vi "Main.vi"(11 "Module Admin":refnum<class "Delacor_lib_QMH_Module Admin.lvclass">) -> ()   [LabVIEW 2022 SP3, in "DBModule.lvlib"]
doc: "This template is based off of the Queued Message Handler design pattern and the Queued Message Handler project template that ships with LabVIEW.\n\nThe main difference is that the queue is private to this module and communication between modules is performed via Broadcast and Request events.\n\nRequest events are wrapped in public API methods and are handled in the Event Handling Loop (EHL) of this VI. Any module can register for Broadcast events sent by this module. The EHL generates messages based on user interface actions.\n\nThe Message Handling Loop (MHL) processes messages generated by the EHL, or by other messages. The messages are string values, so new messages can be added easily to the Message Cases case structure in the MHL. Each message cluster can also provide an optional value for Message Data, which is a variant that can be converted to whatever message-specific data is required.\n____\nHAMPEL SOFTWARE ENGINEERING v2.6.0 (2023-12-19 10:54)"
uses:
  DBModule.lvlib
  <vilib>/Delacor/Delacor QMH/Libraries/Module Admin_class/Delacor_lib_QMH_Module Admin.lvclass
  Module Data--cluster.ctl
  Libraries/hse-libraries/Source/hse-dqmh/Controls/Module Display Scenarios.ctl
  Stop Argument--cluster.ctl
  <vilib>/Delacor/Delacor QMH/Libraries/Message Queue_class/Delacor_lib_QMH_Message Queue.lvclass/Delacor_lib_QMH_Message Queue.ctl
  <vilib>/Delacor/Delacor QMH/Libraries/Module Admin_class/Delacor_lib_QMH_Module Admin.lvclass/Delacor_lib_QMH_Module Admin.ctl
  Configure Argument--cluster.ctl
  Prepare Argument--cluster.ctl
  Request UI Display Argument--cluster.ctl
  Request UI Display (Reply Payload)--cluster.ctl
  Libraries/hse-db/Source/DB-Engines/DB-SQLite/DB-SQLite.lvclass
  C:/Projects/579-Intelligent-Systems-Term-Project/06_Source/UI/FReVSys_Source/Libraries/hse-db/Source/DB-Interface/DB-Interface.lvclass
  <vilib>/Utility/miscctls.llb/LVPointTypeDef.ctl
  <vilib>/Delacor/Delacor QMH/Libraries/Message Queue_class/Delacor_lib_QMH_Enqueue Message (Single).vi
  <vilib>/Delacor/Delacor QMH/Libraries/Module Admin_class/Delacor_lib_QMH_Get External Launch.vi
  <vilib>/Utility/error.llb/Error Cluster From Error Code.vi
  <vilib>/ErrorRing/Error Ring.xnode
  <vilib>/Delacor/Delacor QMH/Libraries/Message Queue_class/Delacor_lib_QMH_Message Queue.lvclass
  Libraries/hse-libraries/Source/hse-configuration/config-ini/config-ini.lvclass
  <vilib>/Hampel Software Engineering/HSE Logger/hse-logger.lvlib
  Libraries/hse-libraries/Source/hse-dqmh/hse-dqmh.lvlib
  Libraries/hse-db/Source/DB_CONNECTOR/DB_CONNECTOR.lvlib
panel:
  in  "Names in DB":string[](array[string])
  in  "Write Names to DB":bool
  in  "Read Names from DB":bool
  out "DB-Engine":string
  out "Status DBC.":string caption="Status of DB_CONNECTOR"
  out "error out":errorcluster
  # "The \"DB Module\" serves as an example of how to use our HSE DB libraries.\n\nThe configuration file of this module (DBModule.ini) points towards the config section to be used in the \nDB_CONNECTOR module's config file (DB_CONNECTOR.ini).\n\nThe module then starts a clone of the DB_CONNECTOR module which it uses to access the SQLite db file.\n\nYou can use the buttons below to read from or write to a `test` table, and the status indicator below re-\ncreates the status display of the DB_CONNECTOR's API tester."
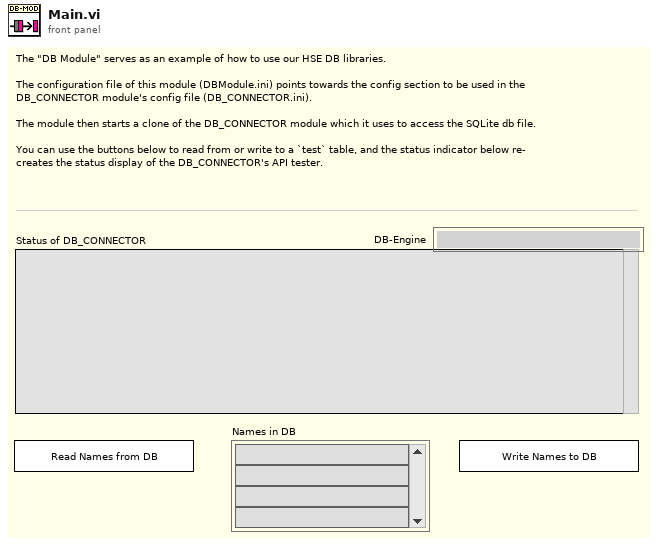
[diagram p1: front panel]
types:
  T1 = typedef "hse-db.lvlib/DB_CONNECTOR.lvlib/Broadcast Events--cluster.ctl" = cluster{"Module Did Init":refnum<user-event>, "Status Updated":refnum<user-event>, "Error Reported":refnum<user-event>, "Module Did Stop":refnum<user-event>, "Update Module Execution Status":refnum<user-event>, "Fast Query Reply":refnum<user-event>, "Configured and Connected":refnum<user-event>}
  T2 = typedef "DBModule.lvlib/Request Events--cluster.ctl" = cluster{"Stop Module":refnum<user-event>, "Show Panel":refnum<user-event>, "Hide Panel":refnum<user-event>, "Get Module Execution Status":refnum<user-event>, "Show Diagram":refnum<user-event>, "Configure":refnum<user-event>, "Prepare":refnum<user-event>, "Request UI Display":refnum<user-event>, "Start and Configure DB_Connector":refnum<user-event>}
  T3 = typedef "DBModule.lvlib/Module Data--cluster.ctl" = cluster{"Scenario":T4, "DB_Connector ID":i32}
  T4 = typedef "hse-dqmh.lvlib/Module Display Scenarios.ctl" = enum16{"Stand-Alone", "Managed"}
  T5 = enum32{"invalid lock state", "Not Locked", "Locked (No Password)", "Password-protected"}
  T6 = typedef "DBModule.lvlib/Stop Argument--cluster.ctl" = cluster{"Origin":string, "Exit via Stop Module Req?":bool, "Wait for Module to stop?":bool}
  T7 = typedef "DBModule.lvlib/Configure Argument--cluster.ctl" = cluster{"Boolean":bool}
  T8 = typedef "DBModule.lvlib/Prepare Argument--cluster.ctl" = cluster{"Boolean":bool}
  T9 = typedef "DBModule.lvlib/Request UI Display Argument--cluster.ctl" = cluster{"Scenario":T4, "Wait Notifier":refnum<notifier>, "wait for reply":bool}
  T10 = typedef "LVPointTypeDef.ctl" = cluster{"Horizontal":i16, "Vertical":i16}
  T11 = enum32{"Invalid", "Standard", "Closed", "Hidden", "Minimized", "Maximized"}
  T12 = typedef "DBModule.lvlib/Request UI Display (Reply Payload)--cluster.ctl" = cluster{"Accept?":bool, "Request UI Display_error":errorcluster}
  T13 = typedef "hse-dqmh.lvlib/System Message Source.ctl" = enum16{"module", "application", "network"}
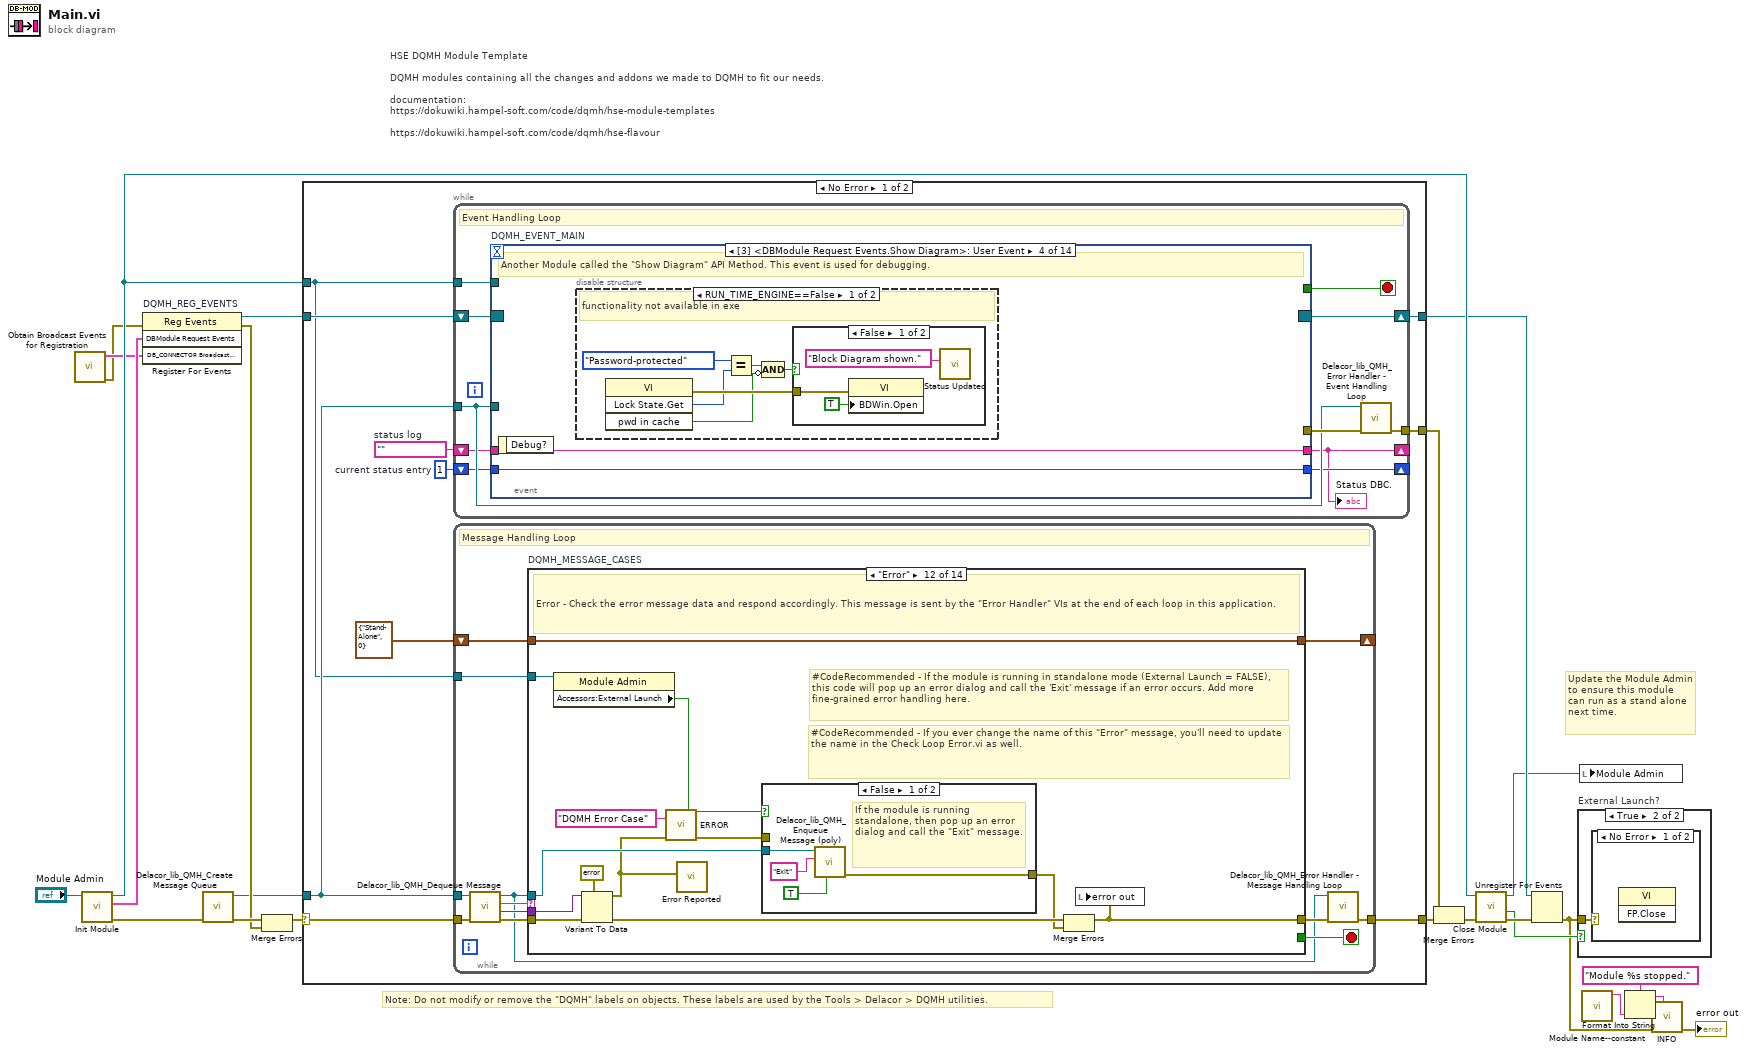
[diagram p0: block diagram]
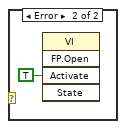
[diagram p3: hidden frame]
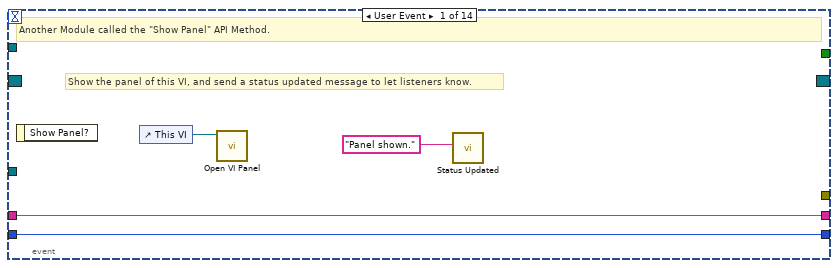
[diagram p4: hidden frame]
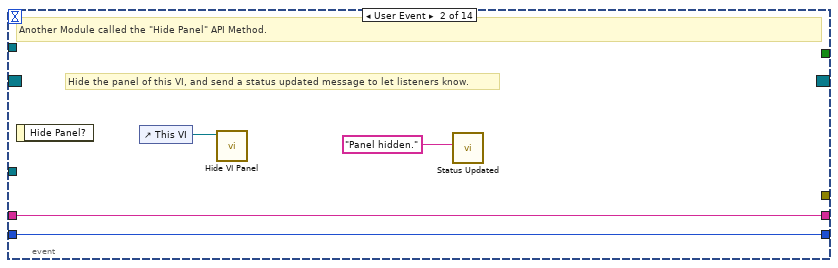
[diagram p5: hidden frame]
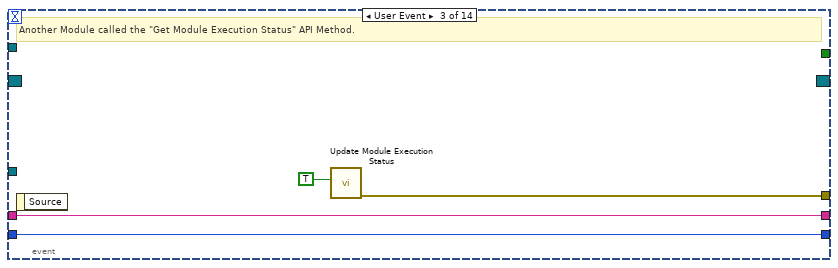
[diagram p6: hidden frame]
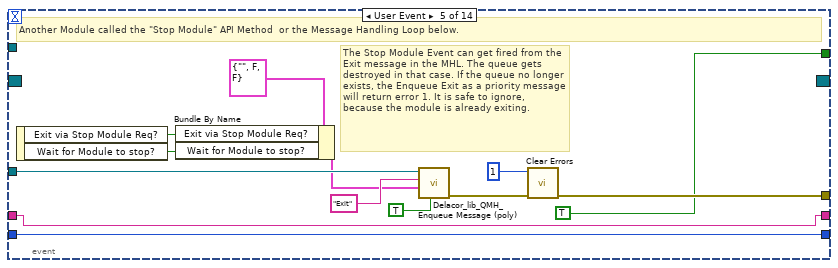
[diagram p9: hidden frame]
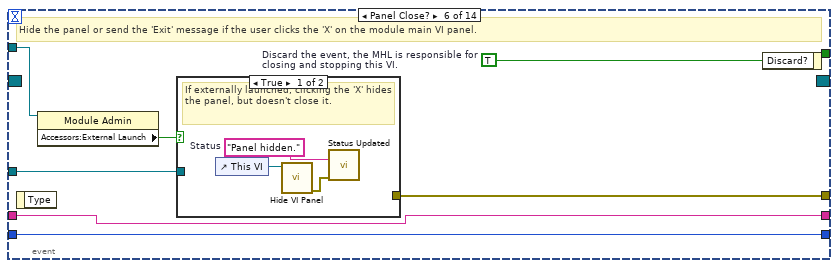
[diagram p10: hidden frame]
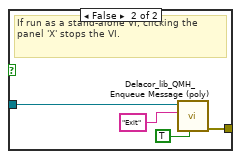
[diagram p11: hidden frame]
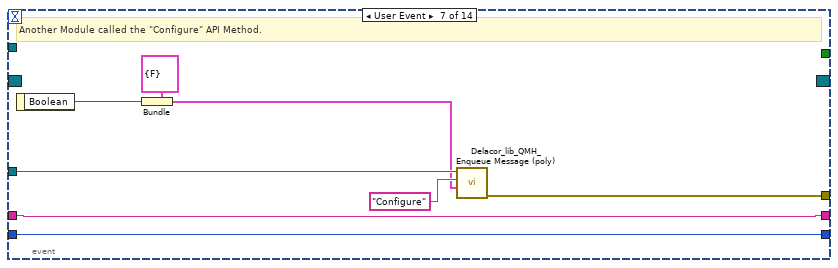
[diagram p12: hidden frame]
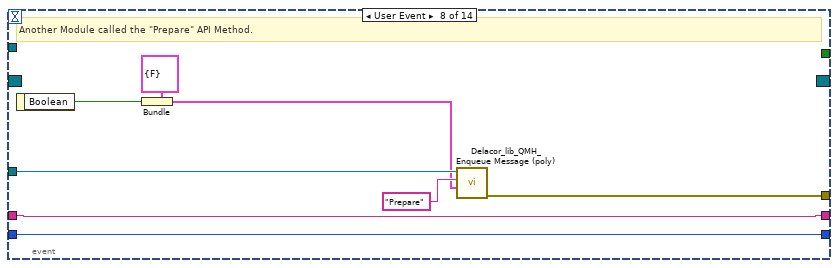
[diagram p13: hidden frame]
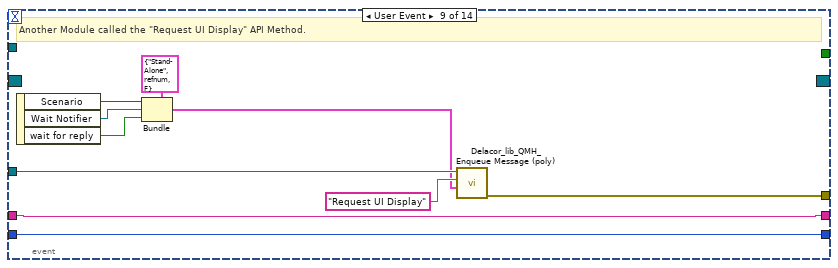
[diagram p14: hidden frame]
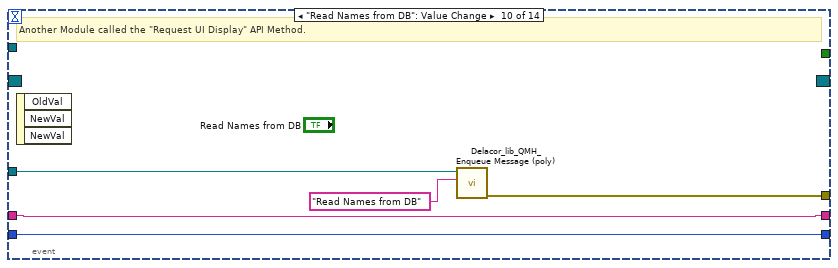
[diagram p15: hidden frame]
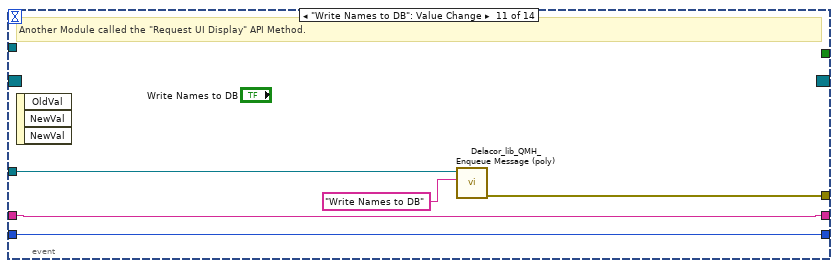
[diagram p16: hidden frame]
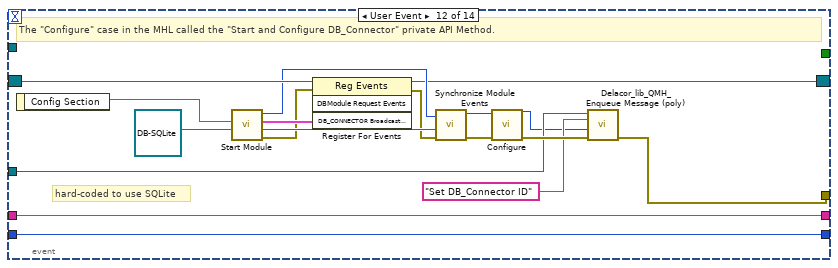
[diagram p17: hidden frame]
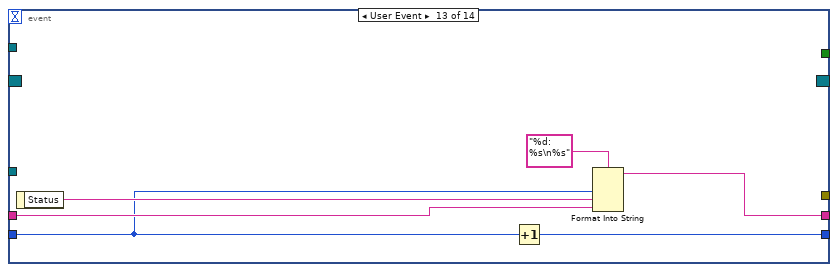
[diagram p18: hidden frame]
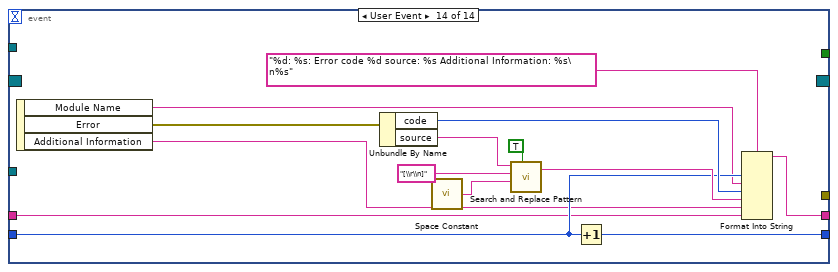
[diagram p19: hidden frame]
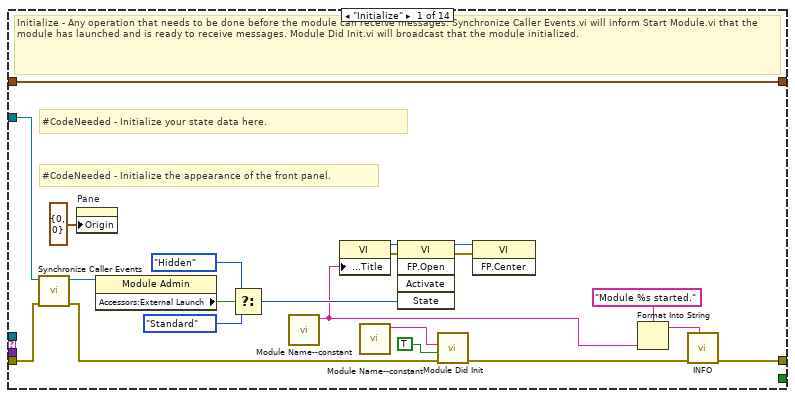
[diagram p20: hidden frame]
diagram:
  # "HSE DQMH Module Template\n\nDQMH modules containing all the changes and addons we made to DQMH to fit our needs.\n\ndocumentation:\nhttps://dokuwiki.hampel-soft.com/code/dqmh/hse-module-templates\n\nhttps://dokuwiki.hampel-soft.com/code/dqmh/hse-flavour"
  # "Note: Do not modify or remove the \"DQMH\" labels on objects. These labels are used by the Tools > Delacor > DQMH utilities."
  # "Update the Module Admin to ensure this module can run as a stand alone next time."
  n1 = call "Obtain Broadcast Events for Registration.vi"() -> ("error out"=w1:errorcluster, "DB_CONNECTOR Broadcast Events"=w2:T1)  [unwired: 10 in]
  n2 = call "Init Module.vi"("Singleton Module Admin in"="Module Admin") -> ("error out"=w22:errorcluster, "DBModule Request Events"=w12:T2, "Singleton Module Admin out"=w15:refnum<class "Delacor_lib_QMH_Module Admin.lvclass">)  [unwired: 8 in]
  n3 = register-events "DQMH_REG_EVENTS"(error in=w1, w12, w2) -> (reference out=w13:refnum<event-registration>, error out=w16:errorcluster)  [unwired: 1 in]
  n4 = call <vilib>:"Delacor_lib_QMH_Create Message Queue.vi"("error in"=w22) -> ("error out"=w18:errorcluster, "Message Queue"=w11:refnum<class "Delacor_lib_QMH_Message Queue.lvclass">)  [unwired: 9 in]
  n5 = Merge Errors(w18, w16) -> (w17:errorcluster)
  n6 = case shown="No Error" w17 {
    selector: w17 -> [w31 w352]
    tunnel: [w33 w352] -> w23
    tunnel: [w30 w349] -> w14
    tunnel: w13 -> [w28 w349]
    tunnel: w11 -> [w27 w344]
    tunnel: [w32 _] -> w20
    tunnel: w15 -> [w26 w345]
    frame No Error {
      w24 = 1  # current status entry
      w25 = ""  # status log
      n7 = while {
        tunnel: w27 -> [w38]
        shift-right: [w41] -> w30
        shift-left: w28 -> [w42]
        tunnel: [w43] -> w32
        tunnel: w26 -> [w39]
        shift-right: [w34] -> _
        shift-left: w25 -> [w37]
        shift-right: [w35] -> _
        shift-left: w24 -> [w36]
        stop <- w40 stop-if-true
        # "Event Handling Loop"
        n8 = event "DQMH_EVENT_MAIN" shown="[3] <DBModule Request Events.Show Diagram>: User Event" {
          selector: w42 -> [_ _ _ _ _ _ _ _ _ _ _ w147 _ _]
          dyn-events: [_ _ _ _ _ _ _ _ _ _ _ w142 _ _] -> w41
          timeout: _ -> [_ _ _ _ _ _ _ _ _ _ _ _ _ _]
          tunnel: [_ _ _ _ TRUE ("Discard?") _ _ _ _ _ _ _ _ _] -> w40
          tunnel: w38 -> [_ _ _ _ w76 w85 w102 w110 w120 w125 w130 w134 _ _]
          tunnel: [_ _ w56 _ w79 w87 w97 w105 w113 w123 w128 w136 _ _] -> w44
          tunnel: w39 -> [_ _ _ _ _ w84 _ _ _ _ _ _ _ _]
          tunnel: w37 -> [w46 w50 w54 w58 w69 w82 w96 w104 w112 w122 w127 w132 w153 w160]
          tunnel: w36 -> [w45 w49 w53 w57 w68 w81 w95 w103 w111 w121 w126 w131 w151 w161]
          tunnel: [w45 w49 w53 w57 w68 w81 w95 w103 w111 w121 w126 w131 w150 w159] -> w35
          tunnel: [w46 w50 w54 w58 w69 w82 w96 w104 w112 w122 w127 w132 w149 w158] -> w34
          event User Event {
            # "Show the panel of this VI, and send a status updated message to let listeners know."
            # "Another Module called the \"Show Panel\" API Method."
            n9 = event-data() -> ()  [unwired: 1 in, 1 out]
            n10 = control-ref of="This VI"() -> (w48:refnum<vi>)
            n11 = call "Open VI Panel.vi"("VI"=w48) -> ()  [unwired: 10 in, 1 out]
            n12 = call "Status Updated.vi"("Status"="Panel shown." ("format string")) -> ()  [unwired: 10 in, 1 out]
          }
          event User Event {
            # "Hide the panel of this VI, and send a status updated message to let listeners know."
            # "Another Module called the \"Hide Panel\" API Method."
            n13 = event-data() -> ()  [unwired: 1 in, 1 out]
            n14 = control-ref of="This VI"() -> (w52:refnum<vi>)
            n15 = call "Hide VI Panel.vi"("VI"=w52) -> ()  [unwired: 10 in, 1 out]
            n16 = call "Status Updated.vi"("Status"="Panel hidden." ("format string")) -> ()  [unwired: 10 in, 1 out]
          }
          event User Event {
            # "Another Module called the \"Get Module Execution Status\" API Method."
            n17 = event-data() -> ()  [unwired: 1 in, 1 out]
            n18 = call "Update Module Execution Status.vi"("Running?"=TRUE) -> ("error out"=w56:errorcluster)  [unwired: 10 in]
          }
          event User Event {
            # "Another Module called the \"Show Diagram\" API Method. This event is used for debugging."
            n19 = event-data() -> ()  [unwired: 1 in, 1 out]
            n20 = disable-structure shown="RUN_TIME_ENGINE==False" {
              frame condition #0 (active) {
                # "functionality not available in exe"
                n21 = invoke on="Invoke Node" class="VI" method="Lock State.Get"() -> (error out=w64:errorcluster, "Get Lock State"=w63:T5, "pwd in cache"=w60:bool)  [unwired: 4 in, 1 out]
                n22 = Equal?(x=T5."Password-protected", y=w63) -> (x = y?=w61:bool)
                n23 = Compound Arithmetic op=AND(w61, invert w60) -> (w59:bool)
                n24 = case shown="False" w59 {
                  tunnel: w64 -> [w67 _]
                  frame False {
                    n25 = property on="Property Node" class="VI"(error in=w67, "BDWin.Open"=TRUE ("Block Diagram Window:Open")) -> ()  [unwired: 1 in, 2 out]
                    n26 = call "Status Updated.vi"("Status"="Block Diagram shown." ("format string")) -> ()  [unwired: 10 in, 1 out]
                  }
                  frame True {
                    # "Password-protected VI, and the password is not in the cache. Do not show the diagram."
                  }
                }
              }
              frame condition #1 {
              }
            }
          }
          event User Event {
            # "The Stop Module Event can get fired from the Exit message in the MHL. The queue gets destroyed in that case. If the queue no longer exists, the Enqueue Exit as a priority message will return error 1. It is safe to ignore, because the module is already exiting."
            # "Another Module called the \"Stop Module\" API Method  or the Message Handling Loop below."
            n27 = event-data() -> ("Exit via Stop Module Req?"=w72:bool, "Wait for Module to stop?"=w71:bool)  [unwired: 1 in]
            n28 = Bundle By Name(cluster=T6 {"Origin"="", "Exit via Stop Module Req?"=FALSE, "Wait for Module to stop?"=FALSE} ("Stop Argument"), "Exit via Stop Module Req?"=w72, "Wait for Module to stop?"=w71) -> (w70:T6)
            n29 = call-poly <vilib>:"Delacor_lib_QMH_Enqueue Message (poly).vi"("Priority Message? (F)"=TRUE, "Message Data"=w70, "Message"="Exit", "Message Queue in"=w76) -> ("error out"=w80:errorcluster)  [unwired: 6 in, 1 out]
            n30 = call <vilib>:"Clear Errors.vi"("error in (no error)"=w80, "specific error code to clear (0: all)"=1) -> ("error out"=w79:errorcluster)  [unwired: 4 in, 1 out]
          }
          event Panel Close? {
            w86 = TRUE  # Discard the event, the MHL is responsible for closing and stopping this VI.
            # "Hide the panel or send the 'Exit' message if the user clicks the 'X' on the module main VI panel."
            n31 = event-data() -> ()  [unwired: 1 in, 1 out]
            n32 = property on="Property Node" class="Module Admin"(reference=w84) -> ("Accessors:External Launch"=w83:bool)  [unwired: 1 in, 2 out]
            n33 = case shown="True" w83 {
              tunnel: w85 -> [_ w93]
              tunnel: [_ w94] -> w87
              frame True {
                w89 = "Panel hidden."  # Status
                # "If externally launched, clicking the 'X' hides the panel, but doesn't close it."
                n34 = control-ref of="This VI"() -> (w90:refnum<vi>)
                n35 = call "Hide VI Panel.vi"("VI"=w90) -> ("error out"=w88:errorcluster)  [unwired: 10 in]
                n36 = call "Status Updated.vi"("error in (no error)"=w88, "Status"=w89) -> ()  [unwired: 9 in, 1 out]
              }
              frame False {
                # "If run as a stand-alone VI, clicking the panel 'X' stops the VI."
                n37 = call-poly <vilib>:"Delacor_lib_QMH_Enqueue Message (poly).vi"("Priority Message? (F)"=TRUE, "Message"="Exit", "Message Queue in"=w93) -> ("error out"=w94:errorcluster)  [unwired: 7 in, 1 out]
              }
            }
            n38 = event-data ("Event Filter Node")("Discard?"=w86) -> ()  [unwired: 1 in, 1 out]
          }
          event User Event {
            # "Another Module called the \"Configure\" API Method."
            n39 = event-data() -> ("Boolean"=w98:bool)  [unwired: 1 in]
            n40 = Bundle(cluster=T7 {"Boolean"=FALSE} ("Configure Argument"), "Boolean"=w98) -> (w99:T7)
            n41 = call-poly <vilib>:"Delacor_lib_QMH_Enqueue Message (poly).vi"("Message Data"=w99, "Message"="Configure", "Message Queue in"=w102) -> ("error out"=w97:errorcluster)  [unwired: 7 in, 1 out]
          }
          event User Event {
            # "Another Module called the \"Prepare\" API Method."
            n42 = event-data() -> ("Boolean"=w106:bool)  [unwired: 1 in]
            n43 = Bundle(cluster=T8 {"Boolean"=FALSE} ("Prepare Argument"), "Boolean"=w106) -> (w107:T8)
            n44 = call-poly <vilib>:"Delacor_lib_QMH_Enqueue Message (poly).vi"("Message Data"=w107, "Message"="Prepare", "Message Queue in"=w110) -> ("error out"=w105:errorcluster)  [unwired: 7 in, 1 out]
          }
          event User Event {
            # "Another Module called the \"Request UI Display\" API Method."
            n45 = event-data() -> ("Scenario"=w116:T4, "Wait Notifier"=w115:refnum<notifier>, "wait for reply"=w114:bool)  [unwired: 1 in]
            n46 = Bundle(cluster=T9 {"Scenario"=enum."Stand-Alone", "Wait Notifier"=refnum, "wait for reply"=FALSE} ("Request UI Display Argument"), "Scenario"=w116, "Wait Notifier"=w115, "wait for reply"=w114) -> (w117:T9)
            n47 = call-poly <vilib>:"Delacor_lib_QMH_Enqueue Message (poly).vi"("Message Data"=w117, "Message"="Request UI Display", "Message Queue in"=w120) -> ("error out"=w113:errorcluster)  [unwired: 7 in, 1 out]
          }
          event "Read Names from DB": Value Change {
            # "Another Module called the \"Request UI Display\" API Method."
            n48 = event-data() -> ()  [unwired: 1 in, 3 out]
            n49 = call-poly <vilib>:"Delacor_lib_QMH_Enqueue Message (poly).vi"("Message"="Read Names from DB", "Message Queue in"=w125) -> ("error out"=w123:errorcluster)  [unwired: 8 in, 1 out]
          }
          event "Write Names to DB": Value Change {
            # "Another Module called the \"Request UI Display\" API Method."
            n50 = event-data() -> ()  [unwired: 1 in, 3 out]
            n51 = call-poly <vilib>:"Delacor_lib_QMH_Enqueue Message (poly).vi"("Message"="Write Names to DB", "Message Queue in"=w130) -> ("error out"=w128:errorcluster)  [unwired: 8 in, 1 out]
          }
          event User Event {
            # "hard-coded to use SQLite"
            # "The \"Configure\" case in the MHL called the \"Start and Configure DB_Connector\" private API Method."
            n52 = event-data() -> ("Config Section"=w145:string)  [unwired: 1 in]
            n53 = call "Start Module.vi"("DB-Engine"=refnum<class "DB-SQLite.lvclass"> refnum ("hse-db-sqlite.lvlib:DB-SQLite"), "Config Section"=w145) -> ("error out"=w139:errorcluster, "Wait for Event Sync?"=w144:bool, "DB_CONNECTOR Broadcast Events"=w146:T1, "Module ID"=w143:i32)  [unwired: 6 in]
            n54 = register-events(reference=w147, error in=w139, w146) -> (reference out=w142:refnum<event-registration>, error out=w138:errorcluster)  [unwired: 1 in]
            n55 = call "Synchronize Module Events.vi"("error in (no error)"=w138, "Wait for Event Sync?"=w144, "Module ID"=w143) -> ("error out"=w140:errorcluster, "Module ID (dup)"=w141:i32)  [unwired: 7 in]
            n56 = call "Configure.vi"("error in (no error)"=w140, "Module ID"=w141) -> ("error out"=w137:errorcluster, "Module ID (dub)"=w133:i32)  [unwired: 8 in]
            n57 = call-poly <vilib>:"Delacor_lib_QMH_Enqueue Message (poly).vi"("error in"=w137, "Message Data"=w133, "Message"="Set DB_Connector ID", "Message Queue in"=w134) -> ("error out"=w136:errorcluster)  [unwired: 6 in, 1 out]
          }
          event User Event {
            n58 = event-data() -> ("Status"=w152:string)  [unwired: 1 in]
            n59 = Increment(x=w151) -> (x+1=w150:i32)
            n60 = Format Into String(format string="%d: %s\n%s", w151, w152, w153) -> (resulting string=w149:string)  [unwired: 2 in, 1 out]
          }
          event User Event {
            n61 = event-data() -> ("Module Name"=w157:string, "Error"=w156:errorcluster, "Additional Information"=w155:string)  [unwired: 1 in]
            n62 = Unbundle By Name(w156) -> ("code"=w163:i32, "source"=w164:string)
            n63 = call <vilib>:"Space Constant.vi"() -> ("String"=w167:string)
            n64 = call <vilib>:"Search and Replace Pattern.vi"("string"=w164, "regular expression (\"\")"="[\\r\\n]" ("regular expression (\"\")"), "replace string (\"\")"=w167, "replace all? (F)"=TRUE ("replace all CR/LF with spaces")) -> ("result string"=w165:string)  [unwired: 1 in, 1 out]
            n65 = Increment(x=w161) -> (x+1=w159:i32)
            n66 = Format Into String(format string="%d: %s: Error code %d source: %s Additional Information: %s\n%s", w161, w157, w163, w165, w155, w160) -> (resulting string=w158:string)  [unwired: 2 in, 1 out]
          }
        }
        "Status DBC." <- w34
        n67 = call-dynamic "Delacor_lib_QMH_Error Handler - Event Handling Loop.vi"("error in"=w44, "Message Queue in"=w38) -> ("dup error in"=w43:errorcluster)  [unwired: 8 in, 1 out]
      }
      n68 = while {
        tunnel: w27 -> [w171]
        shift-right: [w175] -> _
        shift-left: T3 {"Scenario"=enum."Stand-Alone", "DB_Connector ID"=0} ("Data Cluster") -> [w176]
        tunnel: w31 -> [w179]
        tunnel: [w177] -> w33
        tunnel: w26 -> [w169]
        stop <- w174 stop-if-true
        # "Message Handling Loop"
        n69 = call-dynamic "Delacor_lib_QMH_Dequeue Message.vi"("error in"=w179, "Message Queue in"=w171) -> ("error out"=w178:errorcluster, "Message Data"=w172:variant, "Message"=w173:string, "Message Queue out"=w170:refnum<class "Delacor_lib_QMH_Message Queue.lvclass">)  [unwired: 6 in]
        n70 = case "DQMH_MESSAGE_CASES" shown="\"Error\"" w173 {
          selector: w173 -> [_ _ _ _ _ _ _ _ _ _ _ _ _ w331]
          tunnel: w170 -> [_ _ _ w227 _ _ _ _ _ _ _ w299 w323 _]
          tunnel: w178 -> [w199 w203 w209 w238 w244 w258 w267 w272 _ w291 w293 w306 w329 w333]
          tunnel: [w184 w203 w223 w228 w243 w258 w260 w271 w279 w290 w293 w302 w326 w334] -> w180
          tunnel: w176 -> [w190 w202 w213 w232 w247 w257 w266 w275 w282 w289 w292 w301 w315 w332]
          tunnel: [w190 w202 w213 w231 w247 w257 w265 w275 w282 w289 w292 w301 w315 w332] -> w175
          tunnel: [_ _ _ _ _ _ _ _ _ _ _ _ w322 _] -> w174
          tunnel: w172 -> [_ _ _ w237 _ _ w264 _ _ _ _ w300 w321 _]
          tunnel: w169 -> [w191 _ _ _ _ _ _ _ _ _ _ w298 w316 _]
          frame "Initialize" {
            # "#CodeNeeded - Initialize the appearance of the front panel."
            # "#CodeNeeded - Initialize your state data here."
            # "Initialize - Any operation that needs to be done before the module can receive messages. Synchronize Caller Events.vi will inform Start Module.vi that the module has launched and is ready to receive messages. Module Did Init.vi will broadcast that the module initialized."
            n71 = call "Synchronize Caller Events.vi"("error in (no error)"=w199, "Singleton Module Admin in"=w191) -> ("error out"=w198:errorcluster, "Singleton Module Admin out"=w187:refnum<class "Delacor_lib_QMH_Module Admin.lvclass">)  [unwired: 8 in]
            n72 = property on="Pane" class="Pane"("Origin"=T10 {"Horizontal"=0, "Vertical"=0}) -> ()  [unwired: 2 in, 2 out]
            n73 = property on="Property Node" class="Module Admin"(reference=w187) -> ("Accessors:External Launch"=w195:bool)  [unwired: 1 in, 2 out]
            n74 = Select(t=T11."Hidden" ("State"), s=w195, f=T11."Standard" ("State")) -> (s? t:f=w192:T11)
            n75 = call "Module Name--constant.vi"() -> ("Module Name"=w182:string)  [unwired: 11 in]
            n76 = property on="Property Node" class="VI"("Front Panel.Title"=w182) -> (reference out=w197:refnum<vi>, error out=w201:errorcluster)  [unwired: 2 in]
            n77 = call "Module Name--constant.vi"() -> ("Module Name"=w188:string)  [unwired: 11 in]
            n78 = invoke on="Invoke Node" class="VI" method="FP.Open"(reference=w197, error in=w201, "State"=w192) -> (reference out=w196:refnum<vi>, error out=w200:errorcluster)  [unwired: 2 in, 3 out]
            n79 = call "Module Did Init.vi"("error in (no error)"=w198, "Initialized?"=TRUE, "Origin"=w188) -> ("error out"=w185:errorcluster)  [unwired: 8 in]
            n80 = invoke on="Invoke Node" class="VI" method="FP.Center"(reference=w196, error in=w200) -> ()  [unwired: 1 in, 3 out]
            n81 = Format Into String(format string="Module %s started.", w182) -> (resulting string=w181:string)  [unwired: 2 in, 1 out]
            n82 = call <vilib>:"INFO.vi"("Message"=w181, "error in"=w185) -> ("error out"=w184:errorcluster)  [unwired: 9 in]
          }
          frame "---HSE Flavour---" {
            # "Separator -- The following cases handle messages specific to HSE Flavour"
          }
          frame "Configure" {
            w205 = "global" ("Section")
            # "trigger starting the DB_CONNECTOR \nin this module's EHL"
            # "Triggers the auto-configuration of the module."
            n83 = call "Module Name--constant.vi"() -> ("Module Name"=w207:string)  [unwired: 11 in]
            n84 = call "Create Module Config.vi"("error in"=w209, "DQMH Module Name"=w207) -> ("error out"=w208:errorcluster, "config-ini out"=w206:refnum<class "config-ini.lvclass">)  [unwired: 8 in]
            n85 = control-ref of="This VI"() -> (w220:refnum<vi>)
            n86 = call-dynamic "Read String.vi"("Section"=w205, "error in"=w208, "Key"="descriptor" ("Section"), "config-base in"=w206) -> ("error out"=w215:errorcluster, "Value"=w221:string, "config-base out"=w216:refnum<class "config-ini.lvclass">)  [unwired: 5 in]
            n87 = call "DQMH System Message - Add to Run-Time Menu.vi"("Module Descriptor"=w221, "Main VI Reference"=w220) -> ("Payload"=w218:variant, "Identifier"=w217:string, "Source"=w219:T13)  [unwired: 7 in]
            n88 = property on="Property Node" class="VI"("Front Panel.Title"=w221) -> ()  [unwired: 2 in, 2 out]
            n89 = call "System Message.vi"("Sys. Msg. Source"=w219, "Payload"=w218, "Identifier"=w217) -> ()  [unwired: 8 in, 1 out]
            n90 = call-dynamic "Read String.vi"("Section"=w205, "error in"=w215, "Key"="db_connector_config", "config-base in"=w216) -> ("error out"=w211:errorcluster, "Value"=w212:string)  [unwired: 5 in, 1 out]
            n91 = call "Start and Configure DB_Connector.vi"("error in (no error)"=w211, "Config Section"=w212) -> ("error out"=w210:errorcluster)  [unwired: 9 in]
            n92 = call "Module Name--constant.vi"() -> ("Module Name"=w222:string)  [unwired: 11 in]
            n93 = Format Into String(format string="Module %s configured.", w222) -> (resulting string=w224:string)  [unwired: 2 in, 1 out]
            n94 = call <vilib>:"INFO.vi"("Message"=w224, "error in"=w210) -> ("error out"=w223:errorcluster)  [unwired: 9 in]
          }
          frame "Request UI Display" {
            # "#CodeNeeded\n1. Decide if the module can be displayed or not.\n2. Adapt this case accordingly.\n3. Delete or edit this label when done."
            # "Requests the module to display its UI as specified in <b>Scenario</b>:\n\"managed\" => in the UI Manager's subpanel\n\"stand-alone\" => as a separate window"
            n95 = Variant To Data(error in=w238, type=T9 {"Scenario"=enum."Stand-Alone", "Wait Notifier"=refnum, "wait for reply"=FALSE} ("Request UI Display Argument"), Variant=w237) -> (data=w235:T9, error out=w229:errorcluster)
            n96 = Unbundle By Name(w235) -> ("Scenario"=w230:T4, "Wait Notifier"=w234:refnum<notifier>, "wait for reply"=w233:bool)
            n97 = Bundle By Name(cluster=w232, "Scenario"=w230) -> (w231:T3)
            n98 = call-poly <vilib>:"Delacor_lib_QMH_Enqueue Message (poly).vi"("error in"=w229, "Message"="Prepare", "Message Queue in"=w227) -> ("error out"=w228:errorcluster)  [unwired: 7 in, 1 out]
            n99 = case shown="True" w233 {
              tunnel: w234 -> [_ w242]
              frame False {
                # "Without reply."
              }
              frame True {
                # "With reply."
                n100 = Bundle By Name(cluster=T12 {"Accept?"=FALSE, "Request UI Display_error"={"status"=FALSE, "code"=0, "source"=""}} ("Request UI Display (Reply Payload)"), "Accept?"=TRUE) -> (w240:T12)
                n101 = Send Notification(notification=w240, notifier=w242) -> ()  [unwired: 1 in, 2 out]
              }
            }
          }
          frame "Prepare" {
            # "#CodeNeeded\n1. Configure this Message Case for handling the \"Prepare\" message.\n2. Delete or edit this label when done."
            # "Prepare (the UI of the) module for display.\nIn this case  the FP can be updated BEFORE it is shown, if needed."
            n102 = Unbundle By Name(w247) -> ("Scenario"=w246:T4)
            n103 = control-ref of="This VI"() -> (w245:refnum<vi>)
            n104 = case shown="\"Stand-Alone\", Default" w246 {
              tunnel: w245 -> [w248 w253]
              tunnel: w244 -> [w250 w252]
              tunnel: [w249 w251] -> w243
              frame "Stand-Alone", Default {
                n105 = call "Open VI Panel.vi"("error in (no error)"=w250, "VI"=w248) -> ("error out"=w249:errorcluster)  [unwired: 9 in]
              }
              frame "Managed" {
                n106 = call "DQMH System Message - Ready for Display.vi"("Main VI Reference"=w253) -> ("Payload"=w256:variant, "Identifier"=w255:string, "Source"=w254:T13)  [unwired: 8 in]
                n107 = call "System Message.vi"("Sys. Msg. Source"=w254, "error in (no error)"=w252, "Payload"=w256, "Identifier"=w255) -> ("error out"=w251:errorcluster)  [unwired: 7 in]
              }
            }
          }
          frame "--- Module Specific ---" {
            # "Separator -- The following cases handle messages specific to this Module."
          }
          frame "Set DB_Connector ID" {
            n108 = Variant To Data(error in=w267, type=0 ("DB_Connector ID"), Variant=w264) -> (data=w262:i32, error out=w261:errorcluster)
            n109 = call "Get DB-Type.vi"("error in (no error)"=w261, "Module ID"=w262) -> ("error out"=w260:errorcluster, "DB-Type"=→"DB-Engine":string)  [unwired: 8 in]
            n110 = Bundle By Name(cluster=w266, "DB_Connector ID"=w262) -> (w265:T3)
          }
          frame "Read Names from DB" {
            # "read the contents of the table"
            n111 = Unbundle By Name(w275) -> ("DB_Connector ID"=w274:i32)
            n112 = call "Query - String - 2D.vi"("error in"=w272, "Query"="SELECT names FROM test;", "Module ID"=w274) -> ("error out"=w271:errorcluster, "Return Data"=w270:string[][])  [unwired: 5 in, 2 out]
            n113 = Index Array(array=w270, index (col)=0 ("disabled index (col)")) -> (element=w268:string[])  [unwired: 1 in]
            n114 = property on="Names in DB" class="Arr (strict)"("Value"=w268) -> ()  [unwired: 2 in, 2 out]
          }
          frame "Write Names to DB" {
            # "First empty the table, then write the contents of the Listbox back"
            n115 = Unbundle By Name(w282) -> ("DB_Connector ID"=w277:i32)
            n116 = call "Query.vi"("Query"="DELETE FROM test", "Module ID"=w277) -> ("error out"=w276:errorcluster)  [unwired: 7 in, 2 out]
            n117 = for {
              tunnel: "Names in DB" -> [w287] mode=indexing
              tunnel: [w285] -> w280 mode=indexing
              tunnel: w277 -> [w284]
              tunnel: w276 -> [w283]
              n118 = Format Into String(format string="INSERT INTO test (names)\nVALUES ('%s');" ("Query"), w287) -> (resulting string=w286:string)  [unwired: 2 in, 1 out]
              n119 = call "Query.vi"("error in (no error)"=w283, "Query"=w286, "Module ID"=w284) -> ("error out"=w285:errorcluster)  [unwired: 6 in, 2 out]
            }
            n120 = Merge Errors(w280) -> (w279:errorcluster)
          }
          frame "---Copy This Frame---" {
            # "Duplicate this frame when creating new messages.  Change this comment in the duplicated frame to describe this message."
            n121 = Merge Errors(w291) -> (w290:errorcluster)
          }
          frame "--- Exit and Error Handling---" {
            # "Separator - The following cases handle errors and exit messages."
          }
          frame "Error" {
            # "#CodeRecommended - If you ever change the name of this \"Error\" message, you'll need to update the name in the Check Loop Error.vi as well."
            # "#CodeRecommended - If the module is running in standalone mode (External Launch = FALSE), this code will pop up an error dialog and call the 'Exit' message if an error occurs. Add more fine-grained error handling here."
            # "Error - Check the error message data and respond accordingly. This message is sent by the \"Error Handler\" VIs at the end of each loop in this application."
            n122 = property on="Property Node" class="Module Admin"(reference=w298) -> ("Accessors:External Launch"=w297:bool)  [unwired: 1 in, 2 out]
            n123 = Variant To Data(error in=w306, type=errorcluster {"status"=FALSE, "code"=0, "source"=""} ("error constant"), Variant=w300) -> (data=w295:errorcluster, error out=w304:errorcluster)
            n124 = call <vilib>:"ERROR.vi"("Message"="DQMH Error Case", "error in"=w295) -> ("error out"=w294:errorcluster)  [unwired: 9 in]
            n125 = call "Error Reported.vi"("Error"=w295) -> ()  [unwired: 10 in, 1 out]
            n126 = case shown="False" w297 {
              tunnel: [w310 _] -> w303
              tunnel: w299 -> [w309 _]
              tunnel: w294 -> [_ _]
              frame False {
                # "If the module is running standalone, then pop up an error dialog and call the \"Exit\" message."
                n127 = call-poly <vilib>:"Delacor_lib_QMH_Enqueue Message (poly).vi"("Priority Message? (F)"=TRUE, "Message"="Exit", "Message Queue in"=w309) -> ("error out"=w310:errorcluster)  [unwired: 7 in, 1 out]
              }
              frame True {
                # "If the module was launched externally, calling the Error Reported broadcast VI is the only action performed by the \"Error\" message. The module's caller can then process the error appropriately."
              }
            }
            n128 = Merge Errors(w304, w303) -> (w302:errorcluster)
            n129 = local write "error out"(w302) -> ()
          }
          frame "Exit" {
            w320 = 91  # 91: not all Exit messages will have an argument
            w322 = TRUE  # Stop the VI
            # "Release the message queue reference"
            # "#CodeNeeded - Add any required cleanup code here"
            # "Exit - Exit the application."
            n130 = Variant To Data(error in=w329, type=T6 {"Origin"="", "Exit via Stop Module Req?"=FALSE, "Wait for Module to stop?"=FALSE} ("Stop Argument"), Variant=w321) -> (data=w318:T6, error out=w325:errorcluster)
            n131 = call <vilib>:"Clear Errors.vi"("error in (no error)"=w325, "specific error code to clear (0: all)"=w320) -> ("error out"=w328:errorcluster)  [unwired: 4 in, 1 out]
            n132 = control-ref of="This VI"() -> (w317:refnum<vi>)
            n133 = call-dynamic "Delacor_lib_QMH_Release Message Queue.vi"("error in"=w328, "Message Queue"=w323) -> ("error out"=w327:errorcluster)  [unwired: 9 in]
            n134 = call "Handle Exit.vi"("Stop Argument"=w318, "Admin in"=w316, "VI reference"=w317) -> ("error out"=w324:errorcluster)  [unwired: 7 in, 1 out]
            n135 = Unbundle By Name(w315) -> ("DB_Connector ID"=w314:i32)
            n136 = call "Module Name--constant.vi"() -> ("Module Name"=w313:string)  [unwired: 11 in]
            n137 = call "Stop Module.vi"("Wait for Module to stop? (F)"=TRUE, "Origin"=w313, "Module ID"=w314) -> ("error out"=w311:errorcluster)  [unwired: 8 in]
            n138 = Merge Errors(w311, w327, w324) -> (w326:errorcluster)
            n139 = call "Error Reported.vi"("Error"=w326) -> ()  [unwired: 10 in, 1 out]
          }
          frame Default {
            # "'Default' case only runs if there is a message that isn't defined in any of the other cases.  Output a programming error."
            n140 = call "Module Name--constant.vi"() -> ("Module Name"=w330:string)  [unwired: 11 in]
            n141 = xnode "Error Ring"("parameter 0"=w331, "parameter 1"=w330) -> ("error out"=w335:errorcluster)
            n142 = Merge Errors(w333, w335) -> (w334:errorcluster)
          }
        }
        n143 = call-dynamic "Delacor_lib_QMH_Error Handler - Message Handling Loop.vi"("error in"=w180, "Message Queue in"=w170) -> ("dup error in"=w177:errorcluster)  [unwired: 8 in, 1 out]
      }
    }
    frame Error {
      # "Synchronize Caller Events.vi will inform Start Module.vi that the module has launched and will let the code calling Start Module.vi register for broadcasts and would permit the caller receive the broadcast that an error occurred at launch time."
      n144 = call "Synchronize Caller Events.vi"("Singleton Module Admin in"=w345) -> ("error out"=w350:errorcluster)  [unwired: 9 in, 1 out]
      n145 = call-dynamic "Delacor_lib_QMH_Release Message Queue.vi"("Message Queue"=w344) -> ()  [unwired: 10 in, 1 out]
      n146 = call "Module Name--constant.vi"() -> ("Module Name"=w348:string)  [unwired: 11 in]
      n147 = Format Into String(format string="An error occurred during initialization. %s is no longer running.", w348) -> (resulting string=w346:string)  [unwired: 2 in, 1 out]
      n148 = Merge Errors(w352, w350) -> (w351:errorcluster)
      n149 = call "Error Reported.vi"("Additional Information"=w346, "Error"=w351) -> ()  [unwired: 9 in, 1 out]
    }
  }
  n150 = Merge Errors(w20, w23) -> (w19:errorcluster)
  n151 = call "Close Module.vi"("error in (no error)"=w19, "Module Admin in"=w15) -> ("error out"=w21:errorcluster, "External Launch"=w8:bool, "Module Admin out"=w9:refnum<class "Delacor_lib_QMH_Module Admin.lvclass">)  [unwired: 7 in]
  n152 = Unregister For Events(event registration refnum=w14, error in=w21) -> (error out=w5:errorcluster)
  n153 = case "External Launch?" shown="True" w8 {
    tunnel: w5 -> [_ w353]
    frame False {
    }
    frame True {
      n154 = case shown="No Error" w353 {
        frame No Error {
          n155 = invoke on="Invoke Node" class="VI" method="FP.Close"() -> ()  [unwired: 3 in, 3 out]
        }
        frame Error {
          n156 = invoke on="Invoke Node" class="VI" method="FP.Open"("Activate"=TRUE ("Activate?")) -> ()  [unwired: 4 in, 5 out]
        }
      }
    }
  }
  n157 = local write "Module Admin"(w9) -> ()
  n158 = call "Module Name--constant.vi"() -> ("Module Name"=w3:string)  [unwired: 11 in]
  n159 = Format Into String(format string="Module %s stopped.", w3) -> (resulting string=w7:string)  [unwired: 2 in, 1 out]
  n160 = call <vilib>:"INFO.vi"("Message"=w7, "error in"=w5) -> ("error out"=→"error out":errorcluster)  [unwired: 9 in]
